vi "4. Regions of Interest.vi"() -> ()   [LabVIEW 2019]
doc: "c 2020 ReMiSYS All rights reserved."
panel:
  out "ROI":T1
  out "Image Out":T2(plugin-control)
  in  "Stop (F)":bool
  # "1"
  # "2"
  # "3"
  # "4"
  # "5"
  # "6"
  # "7"
  # "10"
  # "11"
  # "12"
  # "1"
  # "1"
  # "2"
  # "2"
  # "3"
  # "3"
  # "12"
  # "10"
  # "4"
  # "5"
  # "c 2022 ReMiSYS All rights reserved."
  # "5"
  # "11"
  # "6"
  # "6"
  # "4"
  # "7"
  # "7"
  # "10"
  # "11"
  # "12"
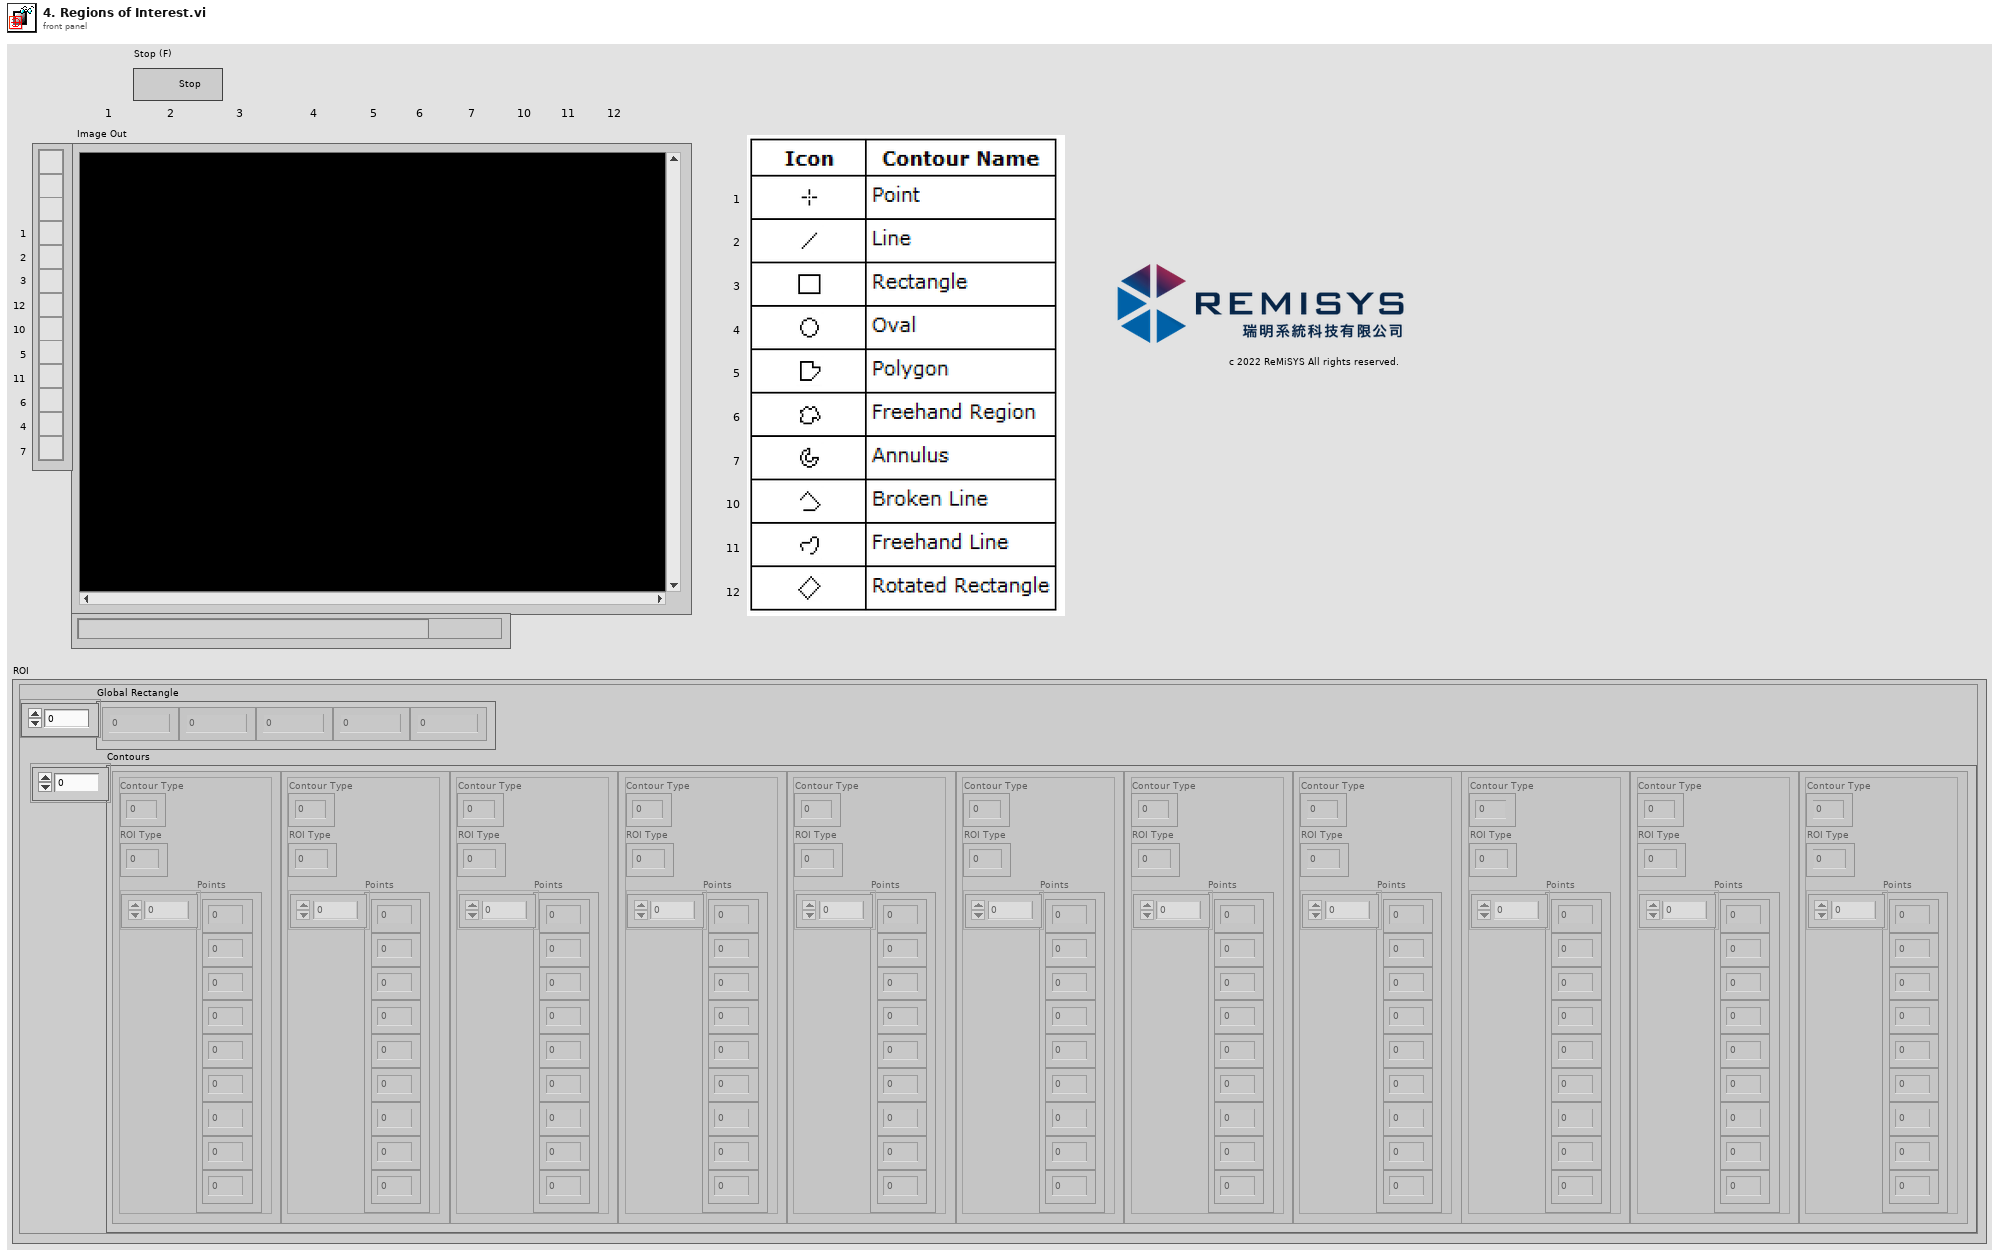
[diagram p1: front panel]
types:
  T1 = cluster{"Global Rectangle":i32[], "Contours":cluster{"Contour Type":u32, "ROI Type":u32, "Points":i32[]}[]}
  T2 = typedef "IMAQ Image.ctl" = refnum<image>
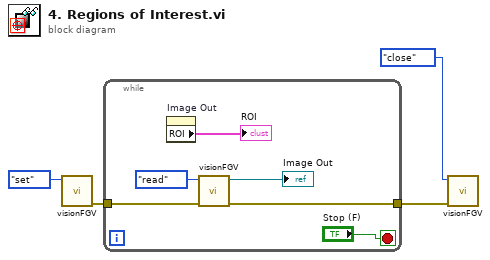
[diagram p0: block diagram]
diagram:
  n1 = call "visionFGV.vi"("Function"=enum16{"set", "read", "close"}."set") -> ("error out"=w3:errorcluster)  [unwired: 9 in, 1 out]
  n2 = while {
    tunnel: w3 -> [w6]
    tunnel: [w5] -> w2
    stop <- "Stop (F)" stop-if-true
    n3 = property on="Image Out" class="ImageControl"() -> ("ROI"=→"ROI":T1)  [unwired: 2 in, 2 out]
    n4 = call "visionFGV.vi"("Error In"=w6, "Function"=enum16{"set", "read", "close"}."read") -> ("error out"=w5:errorcluster, "Image Out fgv"=→"Image Out":T2)  [unwired: 8 in]
  }
  n5 = call "visionFGV.vi"("Error In"=w2, "Function"=enum16{"set", "read", "close"}."close") -> ()  [unwired: 8 in, 2 out]
